vi "3D 曲线.vi"() -> ()   [LabVIEW 2012]
uses:
  <vilib>/Native 3D Graph/xcontrol/3DPC_SurfacePlot.xctl
  <vilib>/imath/engines/lvmath2/RunTimeEngine/ErrorHandling/NIMS_Finalize Error.vi
  <vilib>/imath/engines/lvmath2/RunTimeEngine/NodeEndStatement/NIMS_NodeEndStatement_Output.vi
  <instcachedir>/0/NIMS_NodeEndStatement_Output_53EC0D466D134D7ABD903AC30B43404B.lvgen/NIMS_NodeEndStatement_Output_53EC0D466D134D7ABD903AC30B43404B_005.vi
  <vilib>/imath/engines/lvmath2/RunTimeEngine/BuiltInFunctions/linramp/NIMS_linramp.vi
  <vilib>/imath/engines/lvmath2/RunTimeEngine/BuiltInFunctions/plot3d/NIMS_plot3d.vi
  <vilib>/imathl/engines/lvmath/Functions/Error Handling/Create Error.vi
panel:
  out "3D Graph":refnum<class "Base Datatype.lvclass">[](xcontrol) caption="三维图形"
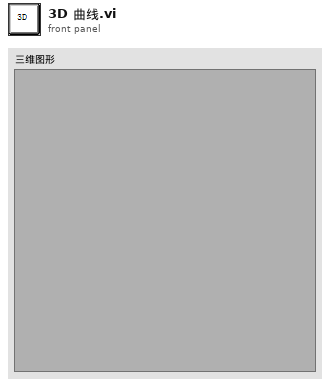
[diagram p1: front panel]
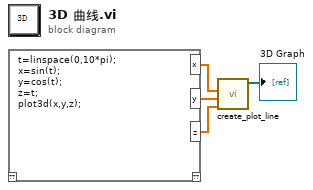
[diagram p0: block diagram]
diagram:
  n1 = mathscript code="t=linspace(0,10*pi);\nx=sin(t);\ny=cos(t);\nz=t;\nplot3d(x,y,z);"() -> ("x"=w3:dbl[], "y"=w2:dbl[], "z"=w1:dbl[])  [unwired: 1 in, 1 out]
  n2 = call <vilib>:"create_plot_line.vi"("z vector"=w1, "y vector"=w2, "x vector"=w3) -> ("plots out"=→"3D Graph":refnum<class "Base Datatype.lvclass">[])  [unwired: 2 in, 6 out]
